vi "FROG_AmplitudePhaseRecover.vi"(4 "Time Array":ext[](array[numeric]), 5 "Signal Array":dbl[](array[numeric])) -> (2 "Array":cluster{ext[], dbl[]}[](array[cluster]))   [LabVIEW 2013]
uses:
  <vilib>/Analysis/2dsp.llb/Complex FFT.vi
  <vilib>/Analysis/NI_AALPro.lvlib
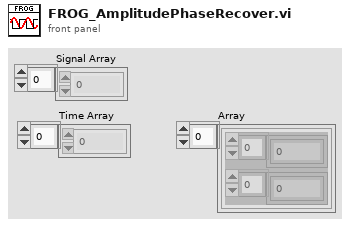
[diagram p1: front panel]
types:
  T1 = cluster{"Time Array":ext[], "Unwrapped Phase":dbl[]}
  T2 = cluster{"Time Array":ext[], "Unwrapped Phase":dbl[]}[]
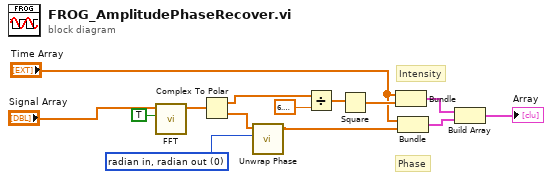
[diagram p0: block diagram]
diagram:
  w6 = 0 items=["radian in, radian out", "radian in, degree out", "degree in, degree out", "degree in, radian out"] ("phase unit")
  # "Intensity"
  # "Phase"
  n1 = call-poly <vilib>:"FFT.vi"("shift?"=TRUE, "X"="Signal Array") -> ("FFT {X}"=w10:cdb[])  [unwired: 8 in, 1 out]
  n2 = Complex To Polar(r * e^(i*theta)=w10) -> (r=w4:dbl[], theta=w7:dbl[])
  n3 = call <vilib>:"Unwrap Phase.vi"("phase unit"=w6, "Phase"=w7) -> ("Unwrapped Phase"=w8:dbl[])  [unwired: 8 in, 1 out]
  n4 = Divide(x=w4, y=6.283185307179586) -> (x/y=w5:dbl[])
  n5 = Square(x=w5) -> (x^2=w11:dbl[])
  n6 = Bundle("Time Array"="Time Array", w11) -> (w12:cluster{"Time Array":ext[], dbl[]})  [unwired: 1 in]
  n7 = Bundle("Time Array"="Time Array", "Unwrapped Phase"=w8) -> (w13:T1)  [unwired: 1 in]
  n8 = Build Array(w12, w13) -> (→"Array":T2)
